vi "1.vi"() -> ()   [LabVIEW 2025, in "2023.lvlib"]
uses:
  2023.lvlib
panel:
  out "sum":i32
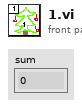
[diagram p1: front panel]
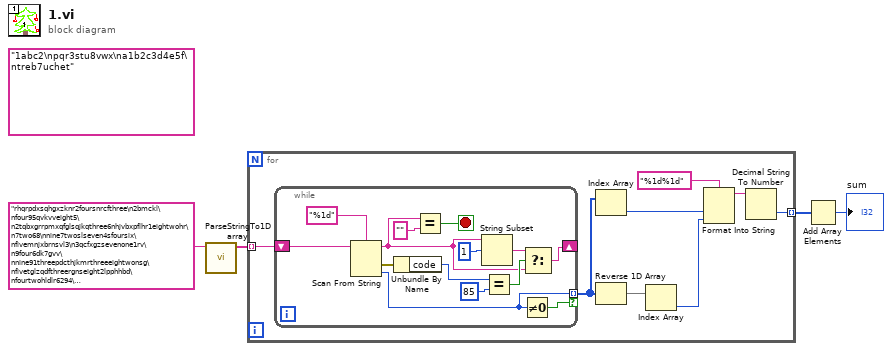
[diagram p0: block diagram]
diagram:
  (unwired) "1abc2\npqr3stu8vwx\na1b2c3d4e5f\ntreb7uchet"
  n1 = call "ParseStringTo1Darray.vi"("Copied Input From Advent Of Code Website"="rhqrpdxsqhgxzknr2foursnrcfthree\n2bmckl\nfour95qvkvveight5\n2tqbxgrrpmxqfglsqjkqthree6nhjvbxpflhr1eightwohr\n7two68\nnine7twoslseven4sfoursix\nfivemnjxbrnsvl3\n3qcfxgzsevenone1rv\n9four6dk7gvv\nnine91threepdcthjkmrthreeeightwonsg\nfivetglzqdfthreergnseight2lpphhbd\nfourtwohldlr6294\nqkvc7pvsv6rvsxlqzpjdjkd1eightthree\nonefourm5qpfvdnbs\nql8jbzzjpsdgmrjtngrkfdmcsix6eightsix\n8nl2\n5lfzqhgeightnine\nthree313eight2zcjnnmtnh\n4three77dgjzfj4five\nntr5sixfourznnljvqdr5one\nthreedlmnd98nineeighteight7\npzcnnbjjthreefmlf9znfnkdrjs\nflbdjkseven7338qxzbcsx6\nsix43fourthree2\none24hndgmz37mjqqm1\n4fiverlgtbr\n7hqtlxgngd15qkfl2th...") -> ("Formatted 1D String Array"=w4:string[])  [unwired: 10 in]
  n2 = for {
    tunnel: w4 -> [w12] mode=indexing
    tunnel: [w5] -> w3 mode=indexing
    n3 = while {
      shift-right: [w15] -> _
      shift-left: w12 -> [w26]
      tunnel: [w14] -> w10 mode=indexing if=w13
      stop <- w23 stop-if-true
      n4 = Scan From String(format string="%1d", input string=w26) -> (remaining string=w16:string, error out=w20:errorcluster, output 1=w14:i32)  [unwired: 3 in, 1 out]
      n5 = Unbundle By Name(w20) -> ("code"=w19:i32)
      n6 = Equal?(x=w16, y="") -> (x = y?=w23:bool)
      n7 = String Subset(string=w16, offset (0)=1) -> (substring=w17:string)  [unwired: 1 in]
      n8 = Equal?(x=w19, y=85 ("number 3")) -> (x = y?=w18:bool)
      n9 = Not Equal To 0?(x=w14) -> (x != 0?=w13:bool)
      n10 = Select(t=w17, s=w18, f=w16) -> (s? t:f=w15:string)
    }
    n11 = Index Array(array=w10) -> (element=w8:i32)  [unwired: 1 in]
    n12 = Reverse 1D Array(array=w10) -> (reversed array=w11:i32[])
    n13 = Index Array(array=w11) -> (element=w7:i32)  [unwired: 1 in]
    n14 = Format Into String(format string="%1d%1d", w8, w7) -> (resulting string=w6:string)  [unwired: 2 in, 1 out]
    n15 = Decimal String To Number(string=w6) -> (number=w5:i32)  [unwired: 2 in, 1 out]
  }
  n16 = Add Array Elements(numeric array=w3) -> (sum=→"sum":i32)
